vi "StateMachineNotesMarcoGonzalez.vi"() -> ()   [LabVIEW 2012]
panel:
  out "Boolean":bool
  out "String":string
  in  "Nickel":bool
  in  "Dime":bool
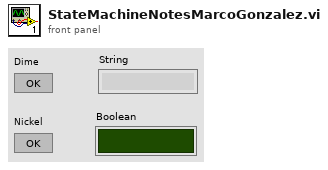
[diagram p1: front panel]
types:
  T1 = enum32{"Start", "5 cents", "10 cents", "Dispense"}
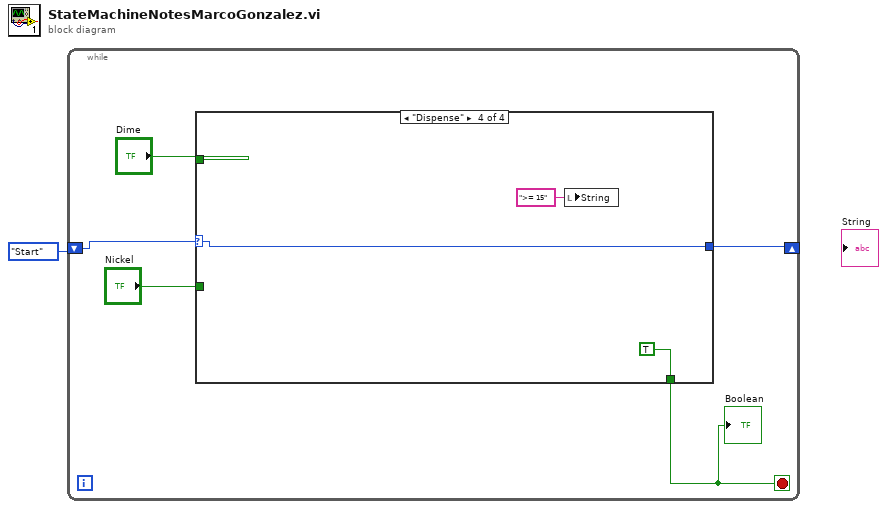
[diagram p0: block diagram]
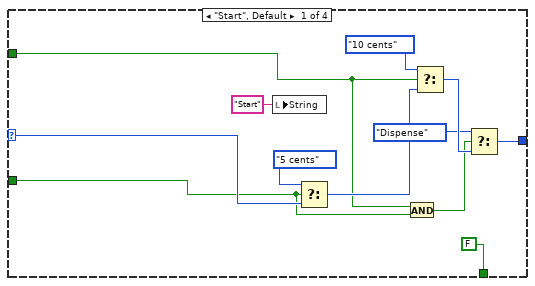
[diagram p2: hidden frame]
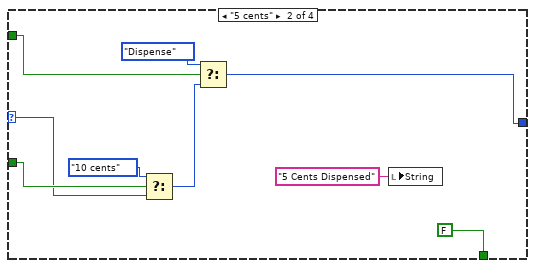
[diagram p3: hidden frame]
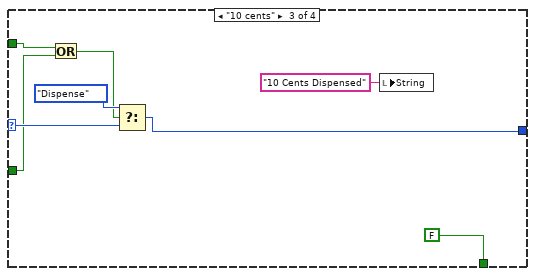
[diagram p4: hidden frame]
diagram:
  n1 = while {
    shift-right: [w3] -> _
    shift-left: T1."Start" -> [w6]
    stop <- w2 stop-if-true
    n2 = case shown="\"Dispense\"" w6 {
      selector: w6 -> [w17 w26 w35 w38]
      tunnel: "Nickel" -> [w11 w27 w33 _]
      tunnel: "Dime" -> [w10 w24 w32 _]
      tunnel: [w12 w21 w30 w38] -> w3
      tunnel: [FALSE FALSE FALSE TRUE] -> w2
      frame "Start", Default {
        n3 = local write "String"("Start" ("String")) -> ()
        n4 = Select(t=T1."5 cents", s=w11, f=w17) -> (s? t:f=w16:T1)
        n5 = And(x=w10, y=w11) -> (x .and. y?=w9:bool)
        n6 = Select(t=T1."10 cents", s=w10, f=w16) -> (s? t:f=w14:T1)
        n7 = Select(t=T1."Dispense", s=w9, f=w14) -> (s? t:f=w12:T1)
      }
      frame "5 cents" {
        n8 = Select(t=T1."10 cents", s=w27, f=w26) -> (s? t:f=w23:T1)
        n9 = Select(t=T1."Dispense", s=w24, f=w23) -> (s? t:f=w21:T1)
        n10 = local write "String"("5 Cents Dispensed" ("String")) -> ()
      }
      frame "10 cents" {
        n11 = Or(x=w32, y=w33) -> (x .or. y?=w31:bool)
        n12 = Select(t=T1."Dispense", s=w31, f=w35) -> (s? t:f=w30:T1)
        n13 = local write "String"("10 Cents Dispensed" ("String")) -> ()
      }
      frame "Dispense" {
        n14 = local write "String"(">= 15" ("String")) -> ()
      }
    }
    "Boolean" <- w2
  }
